vi "Check LIDAR Ranges.vi"(4 "Magnitude":dbl[](array[numeric])) -> (1 "Magnitude out":dbl[](array[numeric]))   [LabVIEW 2018]
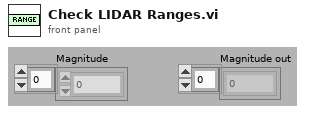
[diagram p1: front panel]
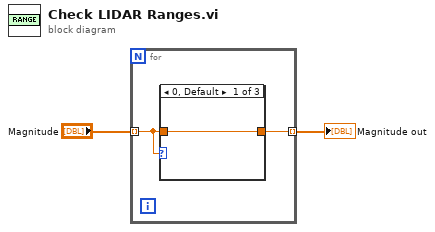
[diagram p0: block diagram]
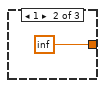
[diagram p2: hidden frame]
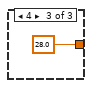
[diagram p3: hidden frame]
diagram:
  n1 = for {
    tunnel: "Magnitude" -> [w4] mode=indexing
    tunnel: [w3] -> w1 mode=indexing
    n2 = case shown="0, Default" w4 {
      tunnel: [w5 inf 28.0 ("Numeric")] -> w3
      tunnel: w4 -> [w5 _ _]
      frame 0, Default {
      }
      frame 1 {
      }
      frame 4 {
      }
    }
  }
  "Magnitude out" <- w1
